vi "NowRT_us.vi"(11 "Error in":errorcluster caption="Error in (no error)") -> (8 "Now":i64 caption="Now [µs]", 15 "Error out":errorcluster)   [LabVIEW 2017, in "GPTiming.lvlib"]
doc: "Returns the current time in <B>Now</B> for use with the RemainingTime and ElapsedTime functions for instance - or if you need a dataflow dependent \"now\" time.\n\nThis VI uses the 32-bit Real-Time microsecond tick counter.\n\nThis VI is inlined. <B>Error in</B> is wired straight through to <B>Error out</B> to enable optional dataflow dependency (offering control of when <B>Now</B> is).\n\nSteen Schmidt\nGPower\n16/12 2013"
uses:
  GPTiming.lvlib
panel:
  # "Copyright © 2013\nGPower\nSee enclosed license file for terms and conditions"
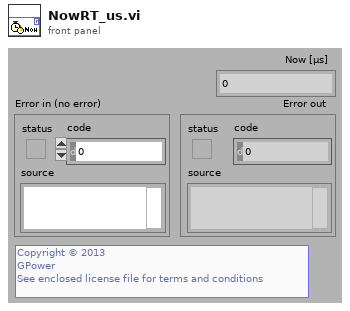
[diagram p1: front panel]
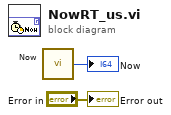
[diagram p0: block diagram]
diagram:
  n1 = call "Now"() -> ("Tick Count(uSec)"=→"Now":u32)
  "Error out" <- "Error in"
